vi "HandleObservationSync_003.vi"(8 "error in (no error)":errorcluster, 11 "S4GUI in":refnum<class "S4GUI.lvclass">) -> (0 "error out":errorcluster, 3 "S4GUI out":refnum<class "S4GUI.lvclass">)   [LabVIEW 2018, in "S4GUI.lvclass"] (continued)
          n765 = call-dynamic "Read AcquisitionC.vi"("error in (no error)"=w1948, "S4ACS_GUI in"=w1947) -> ("error out"=w1927:errorcluster, "Acquisition.lvclass"=w1928:refnum<class "Acquisition.lvclass">, "S4ACS_GUI out"=w1952:refnum<class "S4GUI.lvclass">)  [unwired: 7 in]
          n766 = call "Read connection.vi"("error in (no error)"=w1927, "Server in"=w1928) -> ("error out"=w1926:errorcluster, "connection"=w1924:bool, "Server out"=w1925:refnum<class "Acquisition.lvclass">)  [unwired: 7 in]
          n767 = case shown="True" w1924 {
            tunnel: w1925 -> [w1995 w2011]
            tunnel: w1926 -> [w1994 w2010]
            tunnel: [w1995 w2008] -> w1923
            tunnel: [w1994 w2007] -> w1922
            tunnel: [0 ("State") w1997] -> w1898
            frame False {
            }
            frame True {
              n768 = call-dynamic "Read Channel.vi"("error in (no error)"=w2010, "Acquisition in"=w2011) -> ("error out"=w2006:errorcluster, "Channel.lvclass"=w2005:refnum<class "Channel.lvclass">, "Acquisition out"=w2009:refnum<class "Acquisition.lvclass">)  [unwired: 7 in]
              n769 = call-dynamic "Read State Machine.vi"("error in (no error)"=w2006, "Device in"=w2005) -> ("error out"=w1999:errorcluster, "State Machine.lvclass"=w2001:refnum<class "State Machine.lvclass">, "Device out"=w2003:refnum<class "Channel.lvclass">)  [unwired: 7 in]
              n770 = call-dynamic "Read State.vi"("error in (no error)"=w1999, "State Machine in"=w2001) -> ("error out"=w1998:errorcluster, "State"=w1997:i32, "State Machine out"=w2000:refnum<class "State Machine.lvclass">)  [unwired: 7 in]
              n771 = call-dynamic "Write State Machine.vi"("error in (no error)"=w1998, "State Machine.lvclass"=w2000, "Device in"=w2003) -> ("error out"=w2002:errorcluster, "Device out"=w2004:refnum<class "Channel.lvclass">)  [unwired: 7 in]
              n772 = call-dynamic "Write Channel.vi"("error in (no error)"=w2002, "Channel.lvclass"=w2004, "Acquisition in"=w2009) -> ("error out"=w2007:errorcluster, "Acquisition out"=w2008:refnum<class "Acquisition.lvclass">)  [unwired: 7 in]
            }
          }
          n773 = call-dynamic "Write AcquisitionC.vi"("error in (no error)"=w1922, "Acquisition.lvclass"=w1923, "S4ACS_GUI in"=w1952) -> ("error out"=w1946:errorcluster, "S4ACS_GUI out"=w1945:refnum<class "S4GUI.lvclass">)  [unwired: 7 in]
          n774 = call-dynamic "Read AcquisitionD.vi"("error in (no error)"=w1946, "S4ACS_GUI in"=w1945) -> ("error out"=w1919:errorcluster, "Acquisition.lvclass"=w1921:refnum<class "Acquisition.lvclass">, "S4ACS_GUI out"=w1951:refnum<class "S4GUI.lvclass">)  [unwired: 7 in]
          n775 = call "Read connection.vi"("error in (no error)"=w1919, "Server in"=w1921) -> ("error out"=w1918:errorcluster, "connection"=w1917:bool, "Server out"=w1920:refnum<class "Acquisition.lvclass">)  [unwired: 7 in]
          n776 = case shown="True" w1917 {
            tunnel: w1920 -> [w1977 w1993]
            tunnel: w1918 -> [w1976 w1992]
            tunnel: [w1977 w1990] -> w1916
            tunnel: [w1976 w1989] -> w1915
            tunnel: [0 ("State") w1979] -> w1897
            frame False {
            }
            frame True {
              n777 = call-dynamic "Read Channel.vi"("error in (no error)"=w1992, "Acquisition in"=w1993) -> ("error out"=w1988:errorcluster, "Channel.lvclass"=w1987:refnum<class "Channel.lvclass">, "Acquisition out"=w1991:refnum<class "Acquisition.lvclass">)  [unwired: 7 in]
              n778 = call-dynamic "Read State Machine.vi"("error in (no error)"=w1988, "Device in"=w1987) -> ("error out"=w1981:errorcluster, "State Machine.lvclass"=w1983:refnum<class "State Machine.lvclass">, "Device out"=w1985:refnum<class "Channel.lvclass">)  [unwired: 7 in]
              n779 = call-dynamic "Read State.vi"("error in (no error)"=w1981, "State Machine in"=w1983) -> ("error out"=w1980:errorcluster, "State"=w1979:i32, "State Machine out"=w1982:refnum<class "State Machine.lvclass">)  [unwired: 7 in]
              n780 = call-dynamic "Write State Machine.vi"("error in (no error)"=w1980, "State Machine.lvclass"=w1982, "Device in"=w1985) -> ("error out"=w1984:errorcluster, "Device out"=w1986:refnum<class "Channel.lvclass">)  [unwired: 7 in]
              n781 = call-dynamic "Write Channel.vi"("error in (no error)"=w1984, "Channel.lvclass"=w1986, "Acquisition in"=w1991) -> ("error out"=w1989:errorcluster, "Acquisition out"=w1990:refnum<class "Acquisition.lvclass">)  [unwired: 7 in]
            }
          }
          n782 = call-dynamic "Write AcquisitionD.vi"("error in (no error)"=w1915, "Acquisition.lvclass"=w1916, "S4ACS_GUI in"=w1951) -> ("error out"=w1944:errorcluster, "S4ACS_GUI out"=w1909:refnum<class "S4GUI.lvclass">)  [unwired: 7 in]
          n783 = Equal?(x=w1901, y=w1900) -> (x = y?=w1905:bool)
          n784 = Equal?(x=w1910, y=w1900) -> (x = y?=w1914:bool)
          n785 = Equal?(x=w1901, y=w1899) -> (x = y?=w1904:bool)
          n786 = Equal?(x=w1910, y=w1899) -> (x = y?=w1913:bool)
          n787 = Equal?(x=w1901, y=w1898) -> (x = y?=w1903:bool)
          n788 = Equal?(x=w1910, y=w1898) -> (x = y?=w1912:bool)
          n789 = Equal?(x=w1901, y=w1897) -> (x = y?=w1902:bool)
          n790 = Equal?(x=w1910, y=w1897) -> (x = y?=w1911:bool)
          n791 = Compound Arithmetic op=ADD(w1900, w1899, w1898, w1897) -> (w1908:i32)
          n792 = Compound Arithmetic op=OR(w1905, w1904, w1903, w1902) -> (w1895:bool)
          n793 = Compound Arithmetic op=OR(w1914, w1913, w1912, w1911) -> (w1896:bool)
          n794 = Build Array(w1896, w1895) -> (w1894:bool[])
          n795 = Boolean Array To Number(Boolean array=w1894) -> (number=w1893:u32)
          n796 = case shown="0, Default" w1893 {
            tunnel: w1909 -> [w1959 w1967 w1971 w1975]
            tunnel: [w1958 w1966 w1970 w1974] -> w1906
            tunnel: w1908 -> [w1963 _ _ _]
            tunnel: w1907 -> [w1960 _ _ _]
            frame 0, Default {
              n797 = Equal To 0?(x=w1963) -> (x = 0?=w1962:bool)
              n798 = Select(t=u32 360, s=w1962, f=w1960) -> (s? t:f=w1957:u32)
              n799 = Bundle By Name(cluster=w1959, "Obs_state"=w1957) -> (w1958:refnum<class "S4GUI.lvclass">)
            }
            frame 1 {
              n800 = Bundle By Name(cluster=w1967, "Obs_state"=u32 1, "Error Msg"="ERROR: Some channel initialization failed. S4GUI:HandleObservationSync.vi state 272.") -> (w1966:refnum<class "S4GUI.lvclass">)
            }
            frame 2 {
              n801 = Bundle By Name(cluster=w1971, "Obs_state"=u32 1, "Error Msg"="ERROR: Some channel with invalid Exposition Time. S4GUI:HandleObservationSync.vi state 272.") -> (w1970:refnum<class "S4GUI.lvclass">)
            }
            frame 3 {
              n802 = Bundle By Name(cluster=w1975, "Obs_state"=u32 1, "Error Msg"="ERROR: Invalid configuration in the channels. S4GUI:HandleObservationSync.vi state 272.") -> (w1974:refnum<class "S4GUI.lvclass">)
            }
          }
        }
        frame 299 {
          # "Verifcando iniciação dos CICLO:"
          # "T= todos os canais ativos estão zerados."
          # "Exemplo de erro em \"Cycles_done\":\nchA; cycles_done=0; CCD_STATUS=ACTIVE;                                           Seqs_done=15;\nchA; cycles_done=0; CCD_STATUS=IDLE;                                                Seqs_done=16;   =>mudança de seq. com mesmo ciclo\nchA; cycles_done=1; CCD_STATUS=WAITING_EXPOSE_COMMAND; Seqs_done=0;\n\nchB; cycles_done=0; CCD_STATUS=ACTIVE;                                           Seqs_done=15;\nchB; cycles_done=1; CCD_STATUS=WAITING_EXPOSE_COMMAND; Seqs_done=0;     => mudança de seq com novo ciclo"
          # "T=canais receberam STOP"
          # "T= Todos os canais ativos no mesmo ciclo;\nF= Canais em ciclo diferente."
          # "Todos os CYCLES_DONE \nestão zerados?\nSe sim, vai para 327."
          # "Exemplo:\nSET #CYCLES 3\nSET #SEQ 4\ntotal de sequencias: 3 x 4 = 12\n\nseq.        CYCLES_DONE           SEQS_DONE\n1a.                     0                                 0\n2a.                     0                                 1 \n3a.                     0                                 2 \n4a.                     0                                 3 \n                          1                                 4\n5a.                     1                                 0 \n6a.                     1                                 1 \n7a.                     1                                 2 \n8a.                     1                                 3 \n                          2                                 4\n9a.                     2                                 0 \n10a.                   2                                 1 \n11a.                   2                                 2 \n12a.                   2                                 3 \n\nfim                    3                                 4"
          n803 = call-dynamic "Read AcquisitionA.vi"("error in (no error)"=w2100, "S4ACS_GUI in"=w2066) -> ("error out"=w2081:errorcluster, "Acquisition.lvclass"=w2082:refnum<class "Acquisition.lvclass">, "S4ACS_GUI out"=w2102:refnum<class "S4GUI.lvclass">)  [unwired: 7 in]
          n804 = call-dynamic "Read enabled.vi"("error in (no error)"=w2081, "Server in"=w2082) -> ("error out"=w2080:errorcluster, "enabled"=w2061:bool, "Server out"=w2079:refnum<class "Acquisition.lvclass">)  [unwired: 7 in]
          n805 = case shown="True" w2061 {
            tunnel: w2080 -> [w2192 w2208]
            tunnel: [w2193 w2206] -> w2103
            tunnel: [w2192 w2205] -> w2101
            tunnel: [u32 0 ("SequesDone") w2204] -> _
            tunnel: w2079 -> [w2193 w2203]
            tunnel: [TRUE w2202] -> w2065
            tunnel: [FALSE ("stopping") w2195] -> w2057
            frame False {
            }
            frame True {
              # "CYCLES_DONE = 0 ?"
              n806 = call-dynamic "Read Channel.vi"("error in (no error)"=w2208, "Acquisition in"=w2203) -> ("error out"=w2200:errorcluster, "Channel.lvclass"=w2201:refnum<class "Channel.lvclass">, "Acquisition out"=w2207:refnum<class "Acquisition.lvclass">)  [unwired: 7 in]
              n807 = call-dynamic "Read CyclesDone.vi"("error in (no error)"=w2200, "Channel in"=w2201) -> ("error out"=w2198:errorcluster, "CyclesDone"=w2204:u32, "Channel out"=w2199:refnum<class "Channel.lvclass">)  [unwired: 7 in]
              n808 = Equal?(x=w2204, y=u32 0) -> (x = y?=w2202:bool)
              n809 = call-dynamic "Read stopping.vi"("error in (no error)"=w2198, "Channel in"=w2199) -> ("error out"=w2197:errorcluster, "stopping"=w2195:bool, "Channel out"=w2196:refnum<class "Channel.lvclass">)  [unwired: 7 in]
              n810 = call-dynamic "Write Channel.vi"("error in (no error)"=w2197, "Channel.lvclass"=w2196, "Acquisition in"=w2207) -> ("error out"=w2205:errorcluster, "Acquisition out"=w2206:refnum<class "Acquisition.lvclass">)  [unwired: 7 in]
            }
          }
          n811 = call-dynamic "Write AcquisitionA.vi"("error in (no error)"=w2101, "Acquisition.lvclass"=w2103, "S4ACS_GUI in"=w2102) -> ("error out"=w2098:errorcluster, "S4ACS_GUI out"=w2097:refnum<class "S4GUI.lvclass">)  [unwired: 7 in]
          n812 = call "Read AcquisitionB.vi"("error in (no error)"=w2098, "S4ACS_GUI in"=w2097) -> ("error out"=w2075:errorcluster, "Acquisition.lvclass"=w2078:refnum<class "Acquisition.lvclass">, "S4ACS_GUI out"=w2099:refnum<class "S4GUI.lvclass">)  [unwired: 7 in]
          n813 = call-dynamic "Read enabled.vi"("error in (no error)"=w2075, "Server in"=w2078) -> ("error out"=w2076:errorcluster, "enabled"=w2060:bool, "Server out"=w2077:refnum<class "Acquisition.lvclass">)  [unwired: 7 in]
          n814 = case shown="True" w2060 {
            tunnel: w2076 -> [w2172 w2188]
            tunnel: w2077 -> [w2173 w2187]
            tunnel: [u32 0 ("SequesDone") w2182] -> _
            tunnel: [w2172 w2186] -> w2096
            tunnel: [w2173 w2185] -> w2095
            tunnel: [TRUE w2181] -> w2064
            tunnel: [FALSE ("stopping") w2175] -> w2056
            frame False {
            }
            frame True {
              n815 = call-dynamic "Read Channel.vi"("error in (no error)"=w2188, "Acquisition in"=w2187) -> ("error out"=w2179:errorcluster, "Channel.lvclass"=w2180:refnum<class "Channel.lvclass">, "Acquisition out"=w2183:refnum<class "Acquisition.lvclass">)  [unwired: 7 in]
              n816 = call-dynamic "Read CyclesDone.vi"("error in (no error)"=w2179, "Channel in"=w2180) -> ("error out"=w2177:errorcluster, "CyclesDone"=w2182:u32, "Channel out"=w2184:refnum<class "Channel.lvclass">)  [unwired: 7 in]
              n817 = Equal?(x=w2182, y=u32 0) -> (x = y?=w2181:bool)
              n818 = call-dynamic "Read stopping.vi"("error in (no error)"=w2177, "Channel in"=w2184) -> ("error out"=w2176:errorcluster, "stopping"=w2175:bool, "Channel out"=w2178:refnum<class "Channel.lvclass">)  [unwired: 7 in]
              n819 = call-dynamic "Write Channel.vi"("error in (no error)"=w2176, "Channel.lvclass"=w2178, "Acquisition in"=w2183) -> ("error out"=w2186:errorcluster, "Acquisition out"=w2185:refnum<class "Acquisition.lvclass">)  [unwired: 7 in]
            }
          }
          n820 = call "Write AcquisitionB.vi"("error in (no error)"=w2096, "Acquisition.lvclass"=w2095, "S4ACS_GUI in"=w2099) -> ("error out"=w2088:errorcluster, "S4ACS_GUI out"=w2087:refnum<class "S4GUI.lvclass">)  [unwired: 7 in]
          n821 = call-dynamic "Read AcquisitionC.vi"("error in (no error)"=w2088, "S4ACS_GUI in"=w2087) -> ("error out"=w2072:errorcluster, "Acquisition.lvclass"=w2074:refnum<class "Acquisition.lvclass">, "S4ACS_GUI out"=w2090:refnum<class "S4GUI.lvclass">)  [unwired: 7 in]
          n822 = call-dynamic "Read enabled.vi"("error in (no error)"=w2072, "Server in"=w2074) -> ("error out"=w2071:errorcluster, "enabled"=w2059:bool, "Server out"=w2073:refnum<class "Acquisition.lvclass">)  [unwired: 7 in]
          n823 = case shown="True" w2059 {
            tunnel: [w2152 w2168] -> w2091
            tunnel: [w2153 w2167] -> w2089
            tunnel: w2071 -> [w2152 w2164]
            tunnel: w2073 -> [w2153 w2165]
            tunnel: [u32 0 ("SequesDone") w2163] -> _
            tunnel: [TRUE w2162] -> w2063
            tunnel: [FALSE ("stopping") w2155] -> w2055
            frame False {
            }
            frame True {
              n824 = call-dynamic "Read Channel.vi"("error in (no error)"=w2164, "Acquisition in"=w2165) -> ("error out"=w2159:errorcluster, "Channel.lvclass"=w2160:refnum<class "Channel.lvclass">, "Acquisition out"=w2166:refnum<class "Acquisition.lvclass">)  [unwired: 7 in]
              n825 = call-dynamic "Read CyclesDone.vi"("error in (no error)"=w2159, "Channel in"=w2160) -> ("error out"=w2157:errorcluster, "CyclesDone"=w2163:u32, "Channel out"=w2161:refnum<class "Channel.lvclass">)  [unwired: 7 in]
              n826 = Equal?(x=w2163, y=u32 0) -> (x = y?=w2162:bool)
              n827 = call-dynamic "Read stopping.vi"("error in (no error)"=w2157, "Channel in"=w2161) -> ("error out"=w2156:errorcluster, "stopping"=w2155:bool, "Channel out"=w2158:refnum<class "Channel.lvclass">)  [unwired: 7 in]
              n828 = call-dynamic "Write Channel.vi"("error in (no error)"=w2156, "Channel.lvclass"=w2158, "Acquisition in"=w2166) -> ("error out"=w2168:errorcluster, "Acquisition out"=w2167:refnum<class "Acquisition.lvclass">)  [unwired: 7 in]
            }
          }
          n829 = call-dynamic "Write AcquisitionC.vi"("error in (no error)"=w2091, "Acquisition.lvclass"=w2089, "S4ACS_GUI in"=w2090) -> ("error out"=w2085:errorcluster, "S4ACS_GUI out"=w2086:refnum<class "S4GUI.lvclass">)  [unwired: 7 in]
          n830 = call-dynamic "Read AcquisitionD.vi"("error in (no error)"=w2085, "S4ACS_GUI in"=w2086) -> ("error out"=w2068:errorcluster, "Acquisition.lvclass"=w2070:refnum<class "Acquisition.lvclass">, "S4ACS_GUI out"=w2092:refnum<class "S4GUI.lvclass">)  [unwired: 7 in]
          n831 = call-dynamic "Read enabled.vi"("error in (no error)"=w2068, "Server in"=w2070) -> ("error out"=w2067:errorcluster, "enabled"=w2058:bool, "Server out"=w2069:refnum<class "Acquisition.lvclass">)  [unwired: 7 in]
          n832 = case shown="True" w2058 {
            tunnel: [w2133 w2148] -> w2094
            tunnel: [w2132 w2147] -> w2093
            tunnel: w2069 -> [w2133 w2146]
            tunnel: w2067 -> [w2132 w2145]
            tunnel: [u32 0 ("SequesDone") w2143] -> _
            tunnel: [TRUE w2142] -> w2062
            tunnel: [FALSE ("stopping") w2135] -> w2054
            frame False {
            }
            frame True {
              n833 = call-dynamic "Read Channel.vi"("error in (no error)"=w2145, "Acquisition in"=w2146) -> ("error out"=w2139:errorcluster, "Channel.lvclass"=w2140:refnum<class "Channel.lvclass">, "Acquisition out"=w2144:refnum<class "Acquisition.lvclass">)  [unwired: 7 in]
              n834 = call-dynamic "Read CyclesDone.vi"("error in (no error)"=w2139, "Channel in"=w2140) -> ("error out"=w2137:errorcluster, "CyclesDone"=w2143:u32, "Channel out"=w2141:refnum<class "Channel.lvclass">)  [unwired: 7 in]
              n835 = Equal?(x=w2143, y=u32 0) -> (x = y?=w2142:bool)
              n836 = call-dynamic "Read stopping.vi"("error in (no error)"=w2137, "Channel in"=w2141) -> ("error out"=w2136:errorcluster, "stopping"=w2135:bool, "Channel out"=w2138:refnum<class "Channel.lvclass">)  [unwired: 7 in]
              n837 = call-dynamic "Write Channel.vi"("error in (no error)"=w2136, "Channel.lvclass"=w2138, "Acquisition in"=w2144) -> ("error out"=w2147:errorcluster, "Acquisition out"=w2148:refnum<class "Acquisition.lvclass">)  [unwired: 7 in]
            }
          }
          n838 = Compound Arithmetic op=AND(w2065, w2064, w2063, w2062) -> (w2051:bool)
          n839 = Compound Arithmetic op=OR(w2057, w2056, w2055, w2054) -> (w2053:bool)
          n840 = call-dynamic "Write AcquisitionD.vi"("error in (no error)"=w2093, "Acquisition.lvclass"=w2094, "S4ACS_GUI in"=w2092) -> ("error out"=w2083:errorcluster, "S4ACS_GUI out"=w2084:refnum<class "S4GUI.lvclass">)  [unwired: 7 in]
          n841 = case shown="True" w2051 {
            tunnel: w2084 -> [w2114 w2125]
            tunnel: [w2113 w2124] -> w2052
            tunnel: w2053 -> [_ w2123]
            tunnel: w2050 -> [_ w2120]
            frame False {
              # "Esperando todos os canais habilitados mudarem de cyclesDone.\nE verificando a maior duracao de cubo entre os canais."
              n842 = local read "time307"() -> (w2112:u32)
              n843 = Tick Count (ms)() -> (millisecond timer value=w2111:u32)
              n844 = Subtract(x=w2111, y=w2112) -> (x-y=w2107:u32)
              n845 = call-dynamic "GetGreatestCube.vi"("S4GUI in"=w2114) -> ("S4GUI out"=w2109:refnum<class "S4GUI.lvclass">, "greatest (ms)"=w2105:dbl)  [unwired: 8 in, 1 out]
              n846 = To Double Precision Float(number=w2107) -> (double precision float=w2110:dbl)
              n847 = Add(x=1000.0 ("y"), y=w2105) -> (x+y=w2104:dbl)
              n848 = Less?(x=w2104, y=w2110) -> (x < y?=w2108:bool)
              n849 = case shown="True" w2108 {
                tunnel: w2109 -> [w2115 w2119]
                tunnel: [w2115 w2118] -> w2113
                frame False {
                }
                frame True {
                  n850 = Bundle By Name(cluster=w2119, "Obs_state"=u32 1, "Error Msg"="ERROR: Cycles_Done reseting timeout. - HandleObservationSync.vi state 299.") -> (w2118:refnum<class "S4GUI.lvclass">)
                }
              }
            }
            frame True {
              # "STOP?"
              n851 = case shown="False" w2123 {
                tunnel: [w2126 u32 0] -> w2122
                tunnel: w2120 -> [w2127 _]
                frame False {
                  n852 = Increment(x=w2127) -> (x+1=w2126:u32)
                }
                frame True {
                }
              }
              n853 = Bundle By Name(cluster=w2125, "Obs_state"=w2122, "cyclesDone"=u32 0) -> (w2124:refnum<class "S4GUI.lvclass">)
            }
          }
        }
        frame 300 {
          # "Verifica se é modo fotometria ou polarimetria:\nTrue = polarimetria (esatdo 301)\nFalse = fotometria (estado 321)"
          n854 = flat-sequence {
            tunnel: w2213 -> [w2226]
            tunnel: [w2226] -> w2212
            frame #0 {
              n855 = local read "time3"() -> (w2228:u32)
              n856 = local read "time4"() -> (w2225:u32)
              n857 = Tick Count (ms)() -> (millisecond timer value=w2224:u32)
              n858 = Subtract(x=w2225, y=w2228) -> (x-y=→"delay 3-4":u32)
              n859 = local write "time1"(w2224) -> ()
            }
          }
          n860 = call "Read Instrument.lvclass.vi"("error in (no error)"=w2212, "S4ACS_GUI in"=w2223) -> ("error out"=w2218:errorcluster, "Instrument.lvclass"=w2219:refnum<class "Instrument.lvclass">, "S4ACS_GUI out"=w2217:refnum<class "S4GUI.lvclass">)  [unwired: 7 in]
          n861 = call-dynamic "Read mode.vi"("error in (no error)"=w2218, "Instrument in"=w2219) -> ("error out"=w2214:errorcluster, "mode"=w2216:bool)  [unwired: 7 in, 1 out]
          n862 = Select(t=u32 301, s=w2216, f=u32 321 ("t")) -> (s? t:f=w2221:u32)
          n863 = Bundle By Name(cluster=w2217, "Obs_state"=w2221, "cyclesDone"=u32 0, "sequesDone"=u32 0, "seqAtual"=u32 0) -> (w2222:refnum<class "S4GUI.lvclass">)
        }
        frame 301 {
          # "Configurando para ACS esperar comando EXPOSE"
          n864 = call-dynamic "Read AcquisitionA.vi"("error in (no error)"=w2291, "S4ACS_GUI in"=w2292) -> ("error out"=w2246:errorcluster, "Acquisition.lvclass"=w2247:refnum<class "Acquisition.lvclass">, "S4ACS_GUI out"=w2294:refnum<class "S4GUI.lvclass">)  [unwired: 7 in]
          n865 = call-dynamic "Read enabled.vi"("error in (no error)"=w2246, "Server in"=w2247) -> ("error out"=w2245:errorcluster, "enabled"=w2232:bool, "Server out"=w2248:refnum<class "Acquisition.lvclass">)  [unwired: 7 in]
          n866 = call "Read connection.vi"("error in (no error)"=w2245, "Server in"=w2248) -> ("error out"=w2271:errorcluster, "connection"=w2255:bool, "Server out"=w2272:refnum<class "Acquisition.lvclass">)  [unwired: 7 in]
          n867 = And(x=w2255, y=w2232) -> (x .and. y?=w2256:bool)
          n868 = case shown="True" w2256 {
            tunnel: w2272 -> [w2409 w2428]
            tunnel: w2271 -> [w2408 w2427]
            tunnel: [w2409 w2425] -> w2295
            tunnel: [w2408 w2424] -> w2293
            tunnel: [w2405 u32 0 ("New_State")] -> w2261
            tunnel: w2232 -> [w2404 _]
            frame False {
              n869 = Select(t=u32 1, s=w2404, f=u32 0) -> (s? t:f=w2405:u32)
            }
            frame True {
              n870 = call-dynamic "Read Channel.vi"("error in (no error)"=w2427, "Acquisition in"=w2428) -> ("error out"=w2411:errorcluster, "Channel.lvclass"=w2414:refnum<class "Channel.lvclass">, "Acquisition out"=w2426:refnum<class "Acquisition.lvclass">)  [unwired: 7 in]
              n871 = call-dynamic "Write wait_expose.vi"("error in (no error)"=w2411, "wait_expose"=TRUE, "Channel in"=w2414) -> ("error out"=w2410:errorcluster, "Channel out"=w2413:refnum<class "Channel.lvclass">)  [unwired: 7 in]
              n872 = call-dynamic "Read State Machine.vi"("error in (no error)"=w2410, "Device in"=w2413) -> ("error out"=w2421:errorcluster, "State Machine.lvclass"=w2423:refnum<class "State Machine.lvclass">, "Device out"=w2419:refnum<class "Channel.lvclass">)  [unwired: 7 in]
              n873 = call "Next State.vi"("error in (no error)"=w2421, "New_State"=40, "State Machine in"=w2423) -> ("error out"=w2416:errorcluster, "State Machine out"=w2417:refnum<class "State Machine.lvclass">)  [unwired: 7 in]
              n874 = call-dynamic "Write State Machine.vi"("error in (no error)"=w2416, "State Machine.lvclass"=w2417, "Device in"=w2419) -> ("error out"=w2418:errorcluster, "Device out"=w2420:refnum<class "Channel.lvclass">)  [unwired: 7 in]
              n875 = call-dynamic "Write Channel.vi"("error in (no error)"=w2418, "Channel.lvclass"=w2420, "Acquisition in"=w2426) -> ("error out"=w2424:errorcluster, "Acquisition out"=w2425:refnum<class "Acquisition.lvclass">)  [unwired: 7 in]
            }
          }
          n876 = call-dynamic "Write AcquisitionA.vi"("error in (no error)"=w2293, "Acquisition.lvclass"=w2295, "S4ACS_GUI in"=w2294) -> ("error out"=w2288:errorcluster, "S4ACS_GUI out"=w2289:refnum<class "S4GUI.lvclass">)  [unwired: 7 in]
          n877 = call "Read AcquisitionB.vi"("error in (no error)"=w2288, "S4ACS_GUI in"=w2289) -> ("error out"=w2242:errorcluster, "Acquisition.lvclass"=w2244:refnum<class "Acquisition.lvclass">, "S4ACS_GUI out"=w2286:refnum<class "S4GUI.lvclass">)  [unwired: 7 in]
          n878 = call-dynamic "Read enabled.vi"("error in (no error)"=w2242, "Server in"=w2244) -> ("error out"=w2241:errorcluster, "enabled"=w2231:bool, "Server out"=w2243:refnum<class "Acquisition.lvclass">)  [unwired: 7 in]
          n879 = call "Read connection.vi"("error in (no error)"=w2241, "Server in"=w2243) -> ("error out"=w2269:errorcluster, "connection"=w2253:bool, "Server out"=w2270:refnum<class "Acquisition.lvclass">)  [unwired: 7 in]
          n880 = And(x=w2253, y=w2231) -> (x .and. y?=w2254:bool)
          n881 = case shown="True" w2254 {
            tunnel: w2270 -> [w2384 w2403]
            tunnel: w2269 -> [w2383 w2402]
            tunnel: [w2384 w2400] -> w2287
            tunnel: [w2383 w2399] -> w2285
            tunnel: [w2380 u32 0 ("New_State")] -> w2260
            tunnel: w2231 -> [w2379 _]
            frame False {
              n882 = Select(t=u32 2, s=w2379, f=u32 0) -> (s? t:f=w2380:u32)
            }
            frame True {
              n883 = call-dynamic "Read Channel.vi"("error in (no error)"=w2402, "Acquisition in"=w2403) -> ("error out"=w2386:errorcluster, "Channel.lvclass"=w2388:refnum<class "Channel.lvclass">, "Acquisition out"=w2401:refnum<class "Acquisition.lvclass">)  [unwired: 7 in]
              n884 = call-dynamic "Write wait_expose.vi"("error in (no error)"=w2386, "wait_expose"=TRUE, "Channel in"=w2388) -> ("error out"=w2385:errorcluster, "Channel out"=w2387:refnum<class "Channel.lvclass">)  [unwired: 7 in]
              n885 = call-dynamic "Read State Machine.vi"("error in (no error)"=w2385, "Device in"=w2387) -> ("error out"=w2396:errorcluster, "State Machine.lvclass"=w2398:refnum<class "State Machine.lvclass">, "Device out"=w2394:refnum<class "Channel.lvclass">)  [unwired: 7 in]
              n886 = call "Next State.vi"("error in (no error)"=w2396, "New_State"=40, "State Machine in"=w2398) -> ("error out"=w2391:errorcluster, "State Machine out"=w2392:refnum<class "State Machine.lvclass">)  [unwired: 7 in]
              n887 = call-dynamic "Write State Machine.vi"("error in (no error)"=w2391, "State Machine.lvclass"=w2392, "Device in"=w2394) -> ("error out"=w2393:errorcluster, "Device out"=w2395:refnum<class "Channel.lvclass">)  [unwired: 7 in]
              n888 = call-dynamic "Write Channel.vi"("error in (no error)"=w2393, "Channel.lvclass"=w2395, "Acquisition in"=w2401) -> ("error out"=w2399:errorcluster, "Acquisition out"=w2400:refnum<class "Acquisition.lvclass">)  [unwired: 7 in]
            }
          }
          n889 = call "Write AcquisitionB.vi"("error in (no error)"=w2285, "Acquisition.lvclass"=w2287, "S4ACS_GUI in"=w2286) -> ("error out"=w2281:errorcluster, "S4ACS_GUI out"=w2280:refnum<class "S4GUI.lvclass">)  [unwired: 7 in]
          n890 = call-dynamic "Read AcquisitionC.vi"("error in (no error)"=w2281, "S4ACS_GUI in"=w2280) -> ("error out"=w2238:errorcluster, "Acquisition.lvclass"=w2240:refnum<class "Acquisition.lvclass">, "S4ACS_GUI out"=w2283:refnum<class "S4GUI.lvclass">)  [unwired: 7 in]
          n891 = call-dynamic "Read enabled.vi"("error in (no error)"=w2238, "Server in"=w2240) -> ("error out"=w2237:errorcluster, "enabled"=w2230:bool, "Server out"=w2239:refnum<class "Acquisition.lvclass">)  [unwired: 7 in]
          n892 = call "Read connection.vi"("error in (no error)"=w2237, "Server in"=w2239) -> ("error out"=w2267:errorcluster, "connection"=w2250:bool, "Server out"=w2268:refnum<class "Acquisition.lvclass">)  [unwired: 7 in]
          n893 = And(x=w2250, y=w2230) -> (x .and. y?=w2252:bool)
          n894 = case shown="True" w2252 {
            tunnel: [w2358 w2372] -> w2284
            tunnel: [w2359 w2371] -> w2282
            tunnel: w2268 -> [w2359 w2369]
            tunnel: w2267 -> [w2358 w2368]
            tunnel: [w2355 u32 0 ("New_State")] -> w2259
            tunnel: w2230 -> [w2354 _]
            frame False {
              n895 = Select(t=u32 4, s=w2354, f=u32 0) -> (s? t:f=w2355:u32)
            }
            frame True {
              n896 = call-dynamic "Read Channel.vi"("error in (no error)"=w2368, "Acquisition in"=w2369) -> ("error out"=w2361:errorcluster, "Channel.lvclass"=w2363:refnum<class "Channel.lvclass">, "Acquisition out"=w2370:refnum<class "Acquisition.lvclass">)  [unwired: 7 in]
              n897 = call-dynamic "Write wait_expose.vi"("error in (no error)"=w2361, "wait_expose"=TRUE, "Channel in"=w2363) -> ("error out"=w2360:errorcluster, "Channel out"=w2362:refnum<class "Channel.lvclass">)  [unwired: 7 in]
              n898 = call-dynamic "Read State Machine.vi"("error in (no error)"=w2360, "Device in"=w2362) -> ("error out"=w2375:errorcluster, "State Machine.lvclass"=w2373:refnum<class "State Machine.lvclass">, "Device out"=w2377:refnum<class "Channel.lvclass">)  [unwired: 7 in]
              n899 = call "Next State.vi"("error in (no error)"=w2375, "New_State"=40, "State Machine in"=w2373) -> ("error out"=w2367:errorcluster, "State Machine out"=w2366:refnum<class "State Machine.lvclass">)  [unwired: 7 in]
              n900 = call-dynamic "Write State Machine.vi"("error in (no error)"=w2367, "State Machine.lvclass"=w2366, "Device in"=w2377) -> ("error out"=w2378:errorcluster, "Device out"=w2376:refnum<class "Channel.lvclass">)  [unwired: 7 in]
              n901 = call-dynamic "Write Channel.vi"("error in (no error)"=w2378, "Channel.lvclass"=w2376, "Acquisition in"=w2370) -> ("error out"=w2372:errorcluster, "Acquisition out"=w2371:refnum<class "Acquisition.lvclass">)  [unwired: 7 in]
            }
          }
          n902 = call-dynamic "Write AcquisitionC.vi"("error in (no error)"=w2284, "Acquisition.lvclass"=w2282, "S4ACS_GUI in"=w2283) -> ("error out"=w2278:errorcluster, "S4ACS_GUI out"=w2277:refnum<class "S4GUI.lvclass">)  [unwired: 7 in]
          n903 = call-dynamic "Read AcquisitionD.vi"("error in (no error)"=w2278, "S4ACS_GUI in"=w2277) -> ("error out"=w2234:errorcluster, "Acquisition.lvclass"=w2236:refnum<class "Acquisition.lvclass">, "S4ACS_GUI out"=w2276:refnum<class "S4GUI.lvclass">)  [unwired: 7 in]
          n904 = call-dynamic "Read enabled.vi"("error in (no error)"=w2234, "Server in"=w2236) -> ("error out"=w2233:errorcluster, "enabled"=w2229:bool, "Server out"=w2235:refnum<class "Acquisition.lvclass">)  [unwired: 7 in]
          n905 = call "Read connection.vi"("error in (no error)"=w2233, "Server in"=w2235) -> ("error out"=w2265:errorcluster, "connection"=w2249:bool, "Server out"=w2266:refnum<class "Acquisition.lvclass">)  [unwired: 7 in]
          n906 = And(x=w2249, y=w2229) -> (x .and. y?=w2251:bool)
          n907 = case shown="True" w2251 {
            tunnel: w2265 -> [w2333 w2353]
            tunnel: [w2333 w2352] -> w2279
            tunnel: w2266 -> [w2334 w2345]
            tunnel: [w2334 w2343] -> w2275
            tunnel: [w2330 u32 0 ("New_State")] -> w2258
            tunnel: w2229 -> [w2329 _]
            frame False {
              n908 = Select(t=u32 8, s=w2329, f=u32 0) -> (s? t:f=w2330:u32)
            }
            frame True {
              n909 = call-dynamic "Read Channel.vi"("error in (no error)"=w2353, "Acquisition in"=w2345) -> ("error out"=w2335:errorcluster, "Channel.lvclass"=w2338:refnum<class "Channel.lvclass">, "Acquisition out"=w2344:refnum<class "Acquisition.lvclass">)  [unwired: 7 in]
              n910 = call-dynamic "Write wait_expose.vi"("error in (no error)"=w2335, "wait_expose"=TRUE, "Channel in"=w2338) -> ("error out"=w2336:errorcluster, "Channel out"=w2337:refnum<class "Channel.lvclass">)  [unwired: 7 in]
              n911 = call-dynamic "Read State Machine.vi"("error in (no error)"=w2336, "Device in"=w2337) -> ("error out"=w2349:errorcluster, "State Machine.lvclass"=w2351:refnum<class "State Machine.lvclass">, "Device out"=w2347:refnum<class "Channel.lvclass">)  [unwired: 7 in]
              n912 = call "Next State.vi"("error in (no error)"=w2349, "New_State"=40, "State Machine in"=w2351) -> ("error out"=w2341:errorcluster, "State Machine out"=w2342:refnum<class "State Machine.lvclass">)  [unwired: 7 in]
              n913 = call-dynamic "Write State Machine.vi"("error in (no error)"=w2341, "State Machine.lvclass"=w2342, "Device in"=w2347) -> ("error out"=w2346:errorcluster, "Device out"=w2348:refnum<class "Channel.lvclass">)  [unwired: 7 in]
              n914 = call-dynamic "Write Channel.vi"("error in (no error)"=w2346, "Channel.lvclass"=w2348, "Acquisition in"=w2344) -> ("error out"=w2352:errorcluster, "Acquisition out"=w2343:refnum<class "Acquisition.lvclass">)  [unwired: 7 in]
            }
          }
          n915 = call-dynamic "Write AcquisitionD.vi"("error in (no error)"=w2279, "Acquisition.lvclass"=w2275, "S4ACS_GUI in"=w2276) -> ("error out"=w2274:errorcluster, "S4ACS_GUI out"=w2273:refnum<class "S4GUI.lvclass">)  [unwired: 7 in]
          n916 = Compound Arithmetic op=ADD(w2261, w2260, w2259, w2258) -> (w2262:u32)
          n917 = case shown="0, Default" w2262 {
            tunnel: w2257 -> [w2298 _ _ _ _ _ _ _ _ _ _ _ _ _ _ _]
            tunnel: [w2297 u32 1 ("Obs_state") u32 1 ("Obs_state") u32 1 ("Obs_state") u32 1 ("Obs_state") u32 1 ("Obs_state") u32 1 ("Obs_state") u32 1 ("Obs_state") u32 1 ("Obs_state") u32 1 ("Obs_state") u32 1 ("Obs_state") u32 1 ("Obs_state") u32 1 ("Obs_state") u32 1 ("Obs_state") u32 1 ("Obs_state") u32 1 ("Obs_state")] -> w2263
            tunnel: ["" ("Error Msg") "ERROR: Lost channel 1 connection... - HandleObservationSync.vi state 301" ("Error Msg") "ERROR: Lost channel 2 connection...- HandleObservationSync.vi state 301" ("Error Msg") "ERROR: Lost channels 1 and 2 connection...- HandleObservationSync.vi state 301" ("Error Msg") "ERROR: Lost channel 3 connection...- HandleObservationSync.vi state 301" ("Error Msg") "ERROR: Lost channels 1 and  3 connection...- HandleObservationSync.vi state 301" ("Error Msg") "ERROR:  Lost channels 2 and  3 connection...- HandleObservationSync.vi state 301" ("Error Msg") "ERROR:  Lost channels 1, 2 and  3 connection...- HandleObservationSync.vi state 301" ("Error Msg") "ERROR: Lost channel 4 connection...- HandleObservationSync.vi state 301" ("Error Msg") "ERROR:  Lost channels 1 and 4 connection...- HandleObservationSync.vi state 301" ("Error Msg") "ERROR:  Lost channels 2 and 4 connection...- HandleObservationSync.vi state 301" ("Error Msg") "ERROR: Lost channels 1, 2 and 4 connection...- HandleObservationSync.vi state 301" ("Error Msg") "ERROR: Lost channels 3 and 4 connection...- HandleObservationSync.vi state 301" ("Error Msg") "ERROR: Lost channels 1, 3 and 4 connection...- HandleObservationSync.vi state 301" ("Error Msg") "ERROR: Lost channels 2, 3 and 4 connection...- HandleObservationSync.vi state 301" ("Error Msg") "ERROR: Lost channels 1, 2, 3 and 4 connection...- HandleObservationSync.vi state 301" ("Error Msg")] -> w2264
            frame 0, Default {
              n918 = Increment(x=w2298) -> (x+1=w2297:u32)
            }
            frame 1 {
            }
            frame 2 {
            }
            frame 3 {
            }
            frame 4 {
            }
            frame 5 {
            }
            frame 6 {
            }
            frame 7 {
            }
            frame 8 {
            }
            frame 9 {
            }
            frame 10 {
            }
            frame 11 {
            }
            frame 12 {
            }
            frame 13 {
            }
            frame 14 {
            }
            frame 15 {
            }
          }
          n919 = Bundle By Name(cluster=w2273, "Obs_state"=w2263, "Error Msg"=w2264) -> (w2290:refnum<class "S4GUI.lvclass">)
        }
        frame 302 {
          # "Espera terminar o envio de WAIT EXPOSE COMMAND para todos os ACS."
          n920 = call-dynamic "VerifyAcqIdle.vi"("error in (no error)"=w2430, "S4GUI in"=w2429) -> ("error out"=w2435:errorcluster, "idle"=w2434:bool, "S4GUI out"=w2436:refnum<class "S4GUI.lvclass">)  [unwired: 7 in]
          n921 = Increment(x=w2432) -> (x+1=w2431:u32)
          n922 = Select(t=w2431, s=w2434, f=w2432) -> (s? t:f=w2433:u32)
          n923 = Bundle By Name(cluster=w2436, "Obs_state"=w2433) -> (w2437:refnum<class "S4GUI.lvclass">)
        }
        frame 303 {
          n924 = flat-sequence {
            tunnel: w2443 -> [w2482]
            tunnel: [w2482] -> w2442
            frame #0 {
              n925 = Tick Count (ms)() -> (millisecond timer value=→"time1":u32)
            }
          }
          n926 = call "Read Instrument.lvclass.vi"("error in (no error)"=w2442, "S4ACS_GUI in"=w2478) -> ("error out"=w2480:errorcluster, "Instrument.lvclass"=w2481:refnum<class "Instrument.lvclass">, "S4ACS_GUI out"=w2439:refnum<class "S4GUI.lvclass">)  [unwired: 7 in]
          n927 = call "Read WPROT.vi"("error in (no error)"=w2480, "Instrument in"=w2481) -> ("error out"=w2471:errorcluster, "Opt_Selector.lvclass"=w2472:refnum<class "Opt_Selector.lvclass">, "Instrument out"=w2479:refnum<class "Instrument.lvclass">)  [unwired: 7 in]
          n928 = call-dynamic "getTargetPos.vi"("error in (no error)"=w2471, "Opt_Selector in"=w2472) -> ("error out"=w2470:errorcluster, "Target Pos"=w2450:u16, "Opt_Selector out"=w2469:refnum<class "Opt_Selector.lvclass">)  [unwired: 7 in]
          n929 = Unbundle By Name(w2439) -> ("seqAtual"=w2441:u32)
          n930 = Build Array(-1.0 ("element"), 0.0 ("element"), 22.5 ("element"), 45.0 ("element"), 67.5 ("element"), 90.0 ("element"), 112.5 ("element"), 135.0 ("element"), 157.5 ("element"), 180.0 ("element"), 202.5 ("element"), 225.0 ("element"), 247.5 ("element"), 270.0 ("element"), 292.5 ("element"), 315.0 ("element"), 337.5 ("element")) -> (w2462:dbl[])
          n931 = Index Array(array=w2462, index=w2450) -> (element=w2449:dbl)
          n932 = case shown="0, Default" w2450 {
            selector: w2450 -> [_ w2516]
            tunnel: w2479 -> [w2492 w2504]
            tunnel: [w2492 w2504] -> w2445
            tunnel: [w2489 w2503] -> w2444
            tunnel: w2475 -> [_ w2518]
            tunnel: [u32 314 w2517] -> w2474
            tunnel: w2470 -> [w2490 w2512]
            tunnel: w2469 -> [w2491 w2511]
            tunnel: w2449 -> [_ w2506]
            tunnel: [w2487 w2505] -> w2446
            tunnel: [u32 0 w2494] -> w2440
            tunnel: w2441 -> [_ w2495]
            frame 0, Default {
              # "Terminou uma sequência.\nRecupera as posições em SEQ e desvia para 314 para verificar se há mais ciclos."
              # "Recupera a sequencia anterior para o caso \nde repetição da sequencia (sem precisar clicar \nnas posicoes desejadas novamente)."
              n933 = call-dynamic "Read sequencia_ant.vi"("error in (no error)"=w2490, "Opt_Selector in"=w2491) -> ("error out"=w2486:errorcluster, "sequencia_ant"=w2485:u16, "Opt_Selector out"=w2488:refnum<class "Opt_Selector.lvclass">)  [unwired: 7 in]
              n934 = call-dynamic "Write sequencia.vi"("error in (no error)"=w2486, "sequencia"=w2485, "Opt_Selector in"=w2488) -> ("error out"=w2489:errorcluster, "Opt_Selector out"=w2487:refnum<class "Opt_Selector.lvclass">)  [unwired: 7 in]
            }
            frame 1..16 {
              # "Inicia o Ticks com\nvalor do relogio atual"
              # "Espera até 40 x 0.25s (= 10s) para\nmecanismo entrar em READY"
              n935 = Number To Decimal String(number=w2516) -> (decimal integer string=w2515:string)  [unwired: 1 in]
              n936 = Concatenate Strings("WP" ("string"), w2515) -> (w2513:string)
              n937 = call "Write target name.vi"("error in (no error)"=w2512, "target name"=w2513, "Optics in"=w2511) -> ("error out"=w2509:errorcluster, "Optics out"=w2510:refnum<class "Opt_Selector.lvclass">)  [unwired: 7 in]
              n938 = call "Write target.vi"("error in (no error)"=w2509, "target"=w2506, "Optics in"=w2510) -> ("error out"=w2508:errorcluster, "Optics out"=w2507:refnum<class "Opt_Selector.lvclass">)  [unwired: 7 in]
              n939 = call-dynamic "Read State Machine.vi"("error in (no error)"=w2508, "Device in"=w2507) -> ("error out"=w2520:errorcluster, "State Machine.lvclass"=w2522:refnum<class "State Machine.lvclass">, "Device out"=w2519:refnum<class "Opt_Selector.lvclass">)  [unwired: 7 in]
              n940 = Increment(x=w2518) -> (x+1=w2517:u32)
              n941 = call "Next State.vi"("error in (no error)"=w2520, "New_State"=1, "State Machine in"=w2522) -> ("error out"=w2501:errorcluster, "State Machine out"=w2502:refnum<class "State Machine.lvclass">)  [unwired: 7 in]
              n942 = Increment(x=w2495) -> (x+1=w2494:u32)
              n943 = call-dynamic "Write Timer.vi"("error in (no error)"=w2501, "Timer"=u32 40, "State Machine in"=w2502) -> ("error out"=w2498:errorcluster, "State Machine out"=w2499:refnum<class "State Machine.lvclass">)  [unwired: 7 in]
              n944 = call-dynamic "Init Ticks2.vi"("error in (no error)"=w2498, "State Machine in"=w2499) -> ("error out"=w2497:errorcluster, "State Machine out"=w2496:refnum<class "State Machine.lvclass">)  [unwired: 8 in]
              n945 = call-dynamic "Write State Machine.vi"("error in (no error)"=w2497, "State Machine.lvclass"=w2496, "Device in"=w2519) -> ("error out"=w2503:errorcluster, "Device out"=w2505:refnum<class "Opt_Selector.lvclass">)  [unwired: 7 in]
            }
          }
          n946 = Bundle By Name(cluster=w2439, "seqAtual"=w2440) -> (w2438:refnum<class "S4GUI.lvclass">)
          n947 = call "Write WPROT.vi"("error in (no error)"=w2444, "Opt_Selector.lvclass"=w2446, "Instrument in"=w2445) -> ("error out"=w2448:errorcluster, "Instrument out"=w2447:refnum<class "Instrument.lvclass">)  [unwired: 7 in]
          n948 = call "Write Instrument.lvclass.vi"("error in (no error)"=w2448, "Instrument.lvclass"=w2447, "S4ACS_GUI in"=w2438) -> ("error out"=w2477:errorcluster, "S4ACS_GUI out"=w2476:refnum<class "S4GUI.lvclass">)  [unwired: 7 in]
          n949 = Bundle By Name(cluster=w2476, "Obs_state"=w2474) -> (w2473:refnum<class "S4GUI.lvclass">)
        }
        frame 304 {
          # "Espera terminar o movimento da lamina para disparar a aquisição\ndos canais ativos.\n\nOV 20230424: Não precisa mais atualizar o valor de WPPOS com o\ncomando WRITE_HEADER porque o ACS já recebeu a sequência de\nposições da lâmina."
          n950 = flat-sequence {
            tunnel: w2549 -> [w2574]
            tunnel: [w2574] -> w2548
            frame #0 {
              n951 = Tick Count (ms)() -> (millisecond timer value=w2573:u32)
              "time 2" <- w2573
              n952 = local read "time1"() -> (w2572:u32)
              n953 = Subtract(x=w2573, y=w2572) -> (x-y=→"delay wp":u32)
            }
          }
          n954 = call "Read Instrument.lvclass.vi"("error in (no error)"=w2548, "S4ACS_GUI in"=w2556) -> ("error out"=w2561:errorcluster, "Instrument.lvclass"=w2562:refnum<class "Instrument.lvclass">, "S4ACS_GUI out"=w2558:refnum<class "S4GUI.lvclass">)  [unwired: 7 in]
          n955 = call "Read WPROT.vi"("error in (no error)"=w2561, "Instrument in"=w2562) -> ("error out"=w2555:errorcluster, "Opt_Selector.lvclass"=w2554:refnum<class "Opt_Selector.lvclass">, "Instrument out"=w2560:refnum<class "Instrument.lvclass">)  [unwired: 7 in]
          n956 = call-dynamic "Read State Machine.vi"("error in (no error)"=w2555, "Device in"=w2554) -> ("error out"=w2529:errorcluster, "State Machine.lvclass"=w2532:refnum<class "State Machine.lvclass">, "Device out"=w2552:refnum<class "Opt_Selector.lvclass">)  [unwired: 7 in]
          n957 = call-dynamic "Verif Clock 2.vi"("error in (no error)"=w2529, "period (ms)"=u32 20000 ("period"), "State Machine in"=w2532) -> ("error out"=w2528:errorcluster, "time elapsed"=→"time elapsed":u32, "State Machine out"=w2531:refnum<class "State Machine.lvclass">)  [unwired: 6 in]
          n958 = call-dynamic "Read Timeout 2.vi"("error in (no error)"=w2528, "State Machine in"=w2531) -> ("error out"=w2527:errorcluster, "Timeout 2"=w2535:bool, "State Machine out"=w2530:refnum<class "State Machine.lvclass">)  [unwired: 7 in]
          n959 = call-dynamic "Read State.vi"("error in (no error)"=w2527, "State Machine in"=w2530) -> ("error out"=w2546:errorcluster, "State"=w2550:i32, "State Machine out"=w2547:refnum<class "State Machine.lvclass">)  [unwired: 7 in]
          n960 = Equal To 0?(x=w2550) -> (x = 0?=w2538:bool)
          n961 = call-dynamic "Write State Machine.vi"("error in (no error)"=w2546, "State Machine.lvclass"=w2547, "Device in"=w2552) -> ("error out"=w2551:errorcluster, "Device out"=w2553:refnum<class "Opt_Selector.lvclass">)  [unwired: 7 in]
          n962 = call "Write WPROT.vi"("error in (no error)"=w2551, "Opt_Selector.lvclass"=w2553, "Instrument in"=w2560) -> ("error out"=w2557:errorcluster, "Instrument out"=w2559:refnum<class "Instrument.lvclass">)  [unwired: 7 in]
          n963 = call "Write Instrument.lvclass.vi"("error in (no error)"=w2557, "Instrument.lvclass"=w2559, "S4ACS_GUI in"=w2558) -> ("error out"=w2537:errorcluster, "S4ACS_GUI out"=w2526:refnum<class "S4GUI.lvclass">)  [unwired: 7 in]
          n964 = case shown="True" w2535 {
            tunnel: w2534 -> [w2564 _]
            tunnel: [w2564 u32 1 ("Obs_state")] -> w2533
            tunnel: w2526 -> [w2563 w2568]
            tunnel: [w2563 w2567] -> w2525
            frame False {
            }
            frame True {
              n965 = Bundle By Name(cluster=w2568, "Error Msg"="ERROR: moving waveplate timeout  (S4GUI:HandleObservationSync.vi - state 302)") -> (w2567:refnum<class "S4GUI.lvclass">)
            }
          }
          n966 = Unbundle By Name(w2526) -> ("cyclesDone"=w2542:u32, "seqAtual"=w2541:u32)
          n967 = Decrement(x=w2541) -> (x-1=w2523:u32)
          n968 = Add(x=w2542, y=w2523) -> (x+y=w2540:u32)
          n969 = Equal To 0?(x=w2540) -> (x = 0?=w2543:bool)
          n970 = case shown="True" w2543 {
            tunnel: [u32 308 ("t") u32 308 ("t")] -> w2544
            frame False {
              (unwired) u32 310 ("t")
              # "Não é 1a seq:\nvai direto para\nenvio do trigger"
            }
            frame True {
              # "1a sequencia:\nenvia EXPOSE"
            }
          }
          n971 = Select(t=w2544, s=w2538, f=w2533) -> (s? t:f=w2545:u32)
          n972 = Bundle By Name(cluster=w2525, "Obs_state"=w2545) -> (w2539:refnum<class "S4GUI.lvclass">)
        }
        frame 308 {
          n973 = call-dynamic "Read AcquisitionA.vi"("error in (no error)"=w2637, "S4ACS_GUI in"=w2638) -> ("error out"=w2592:errorcluster, "Acquisition.lvclass"=w2593:refnum<class "Acquisition.lvclass">, "S4ACS_GUI out"=w2640:refnum<class "S4GUI.lvclass">)  [unwired: 7 in]
          n974 = call-dynamic "Read enabled.vi"("error in (no error)"=w2592, "Server in"=w2593) -> ("error out"=w2591:errorcluster, "enabled"=w2578:bool, "Server out"=w2594:refnum<class "Acquisition.lvclass">)  [unwired: 7 in]
          n975 = call "Read connection.vi"("error in (no error)"=w2591, "Server in"=w2594) -> ("error out"=w2617:errorcluster, "connection"=w2601:bool, "Server out"=w2618:refnum<class "Acquisition.lvclass">)  [unwired: 7 in]
          n976 = And(x=w2601, y=w2578) -> (x .and. y?=w2602:bool)
          n977 = case shown="True" w2602 {
            tunnel: w2618 -> [w2747 w2763]
            tunnel: w2617 -> [w2746 w2762]
            tunnel: [w2747 w2760] -> w2641
            tunnel: [w2746 w2759] -> w2639
            tunnel: [w2743 u32 0 ("New_State")] -> w2607
            tunnel: w2578 -> [w2742 _]
            frame False {
              n978 = Select(t=u32 1, s=w2742, f=u32 0) -> (s? t:f=w2743:u32)
            }
            frame True {
              n979 = call-dynamic "Read Channel.vi"("error in (no error)"=w2762, "Acquisition in"=w2763) -> ("error out"=w2755:errorcluster, "Channel.lvclass"=w2754:refnum<class "Channel.lvclass">, "Acquisition out"=w2761:refnum<class "Acquisition.lvclass">)  [unwired: 7 in]
              n980 = call-dynamic "Read State Machine.vi"("error in (no error)"=w2755, "Device in"=w2754) -> ("error out"=w2756:errorcluster, "State Machine.lvclass"=w2758:refnum<class "State Machine.lvclass">, "Device out"=w2752:refnum<class "Channel.lvclass">)  [unwired: 7 in]
              n981 = call "Next State.vi"("error in (no error)"=w2756, "New_State"=50, "State Machine in"=w2758) -> ("error out"=w2749:errorcluster, "State Machine out"=w2750:refnum<class "State Machine.lvclass">)  [unwired: 7 in]
              n982 = call-dynamic "Write State Machine.vi"("error in (no error)"=w2749, "State Machine.lvclass"=w2750, "Device in"=w2752) -> ("error out"=w2751:errorcluster, "Device out"=w2753:refnum<class "Channel.lvclass">)  [unwired: 7 in]
              n983 = call-dynamic "Write Channel.vi"("error in (no error)"=w2751, "Channel.lvclass"=w2753, "Acquisition in"=w2761) -> ("error out"=w2759:errorcluster, "Acquisition out"=w2760:refnum<class "Acquisition.lvclass">)  [unwired: 7 in]
            }
          }
          n984 = call-dynamic "Write AcquisitionA.vi"("error in (no error)"=w2639, "Acquisition.lvclass"=w2641, "S4ACS_GUI in"=w2640) -> ("error out"=w2634:errorcluster, "S4ACS_GUI out"=w2635:refnum<class "S4GUI.lvclass">)  [unwired: 7 in]
          n985 = call "Read AcquisitionB.vi"("error in (no error)"=w2634, "S4ACS_GUI in"=w2635) -> ("error out"=w2588:errorcluster, "Acquisition.lvclass"=w2590:refnum<class "Acquisition.lvclass">, "S4ACS_GUI out"=w2632:refnum<class "S4GUI.lvclass">)  [unwired: 7 in]
          n986 = call-dynamic "Read enabled.vi"("error in (no error)"=w2588, "Server in"=w2590) -> ("error out"=w2587:errorcluster, "enabled"=w2577:bool, "Server out"=w2589:refnum<class "Acquisition.lvclass">)  [unwired: 7 in]
          n987 = call "Read connection.vi"("error in (no error)"=w2587, "Server in"=w2589) -> ("error out"=w2615:errorcluster, "connection"=w2599:bool, "Server out"=w2616:refnum<class "Acquisition.lvclass">)  [unwired: 7 in]
          n988 = And(x=w2599, y=w2577) -> (x .and. y?=w2600:bool)
          n989 = case shown="True" w2600 {
            tunnel: w2616 -> [w2725 w2741]
            tunnel: w2615 -> [w2724 w2740]
            tunnel: [w2725 w2738] -> w2633
            tunnel: [w2724 w2737] -> w2631
            tunnel: [w2721 u32 0 ("New_State")] -> w2606
            tunnel: w2577 -> [w2720 _]
            frame False {
              n990 = Select(t=u32 2, s=w2720, f=u32 0) -> (s? t:f=w2721:u32)
            }
            frame True {
              n991 = call-dynamic "Read Channel.vi"("error in (no error)"=w2740, "Acquisition in"=w2741) -> ("error out"=w2733:errorcluster, "Channel.lvclass"=w2732:refnum<class "Channel.lvclass">, "Acquisition out"=w2739:refnum<class "Acquisition.lvclass">)  [unwired: 7 in]
              n992 = call-dynamic "Read State Machine.vi"("error in (no error)"=w2733, "Device in"=w2732) -> ("error out"=w2734:errorcluster, "State Machine.lvclass"=w2736:refnum<class "State Machine.lvclass">, "Device out"=w2730:refnum<class "Channel.lvclass">)  [unwired: 7 in]
              n993 = call "Next State.vi"("error in (no error)"=w2734, "New_State"=50, "State Machine in"=w2736) -> ("error out"=w2727:errorcluster, "State Machine out"=w2728:refnum<class "State Machine.lvclass">)  [unwired: 7 in]
              n994 = call-dynamic "Write State Machine.vi"("error in (no error)"=w2727, "State Machine.lvclass"=w2728, "Device in"=w2730) -> ("error out"=w2729:errorcluster, "Device out"=w2731:refnum<class "Channel.lvclass">)  [unwired: 7 in]
              n995 = call-dynamic "Write Channel.vi"("error in (no error)"=w2729, "Channel.lvclass"=w2731, "Acquisition in"=w2739) -> ("error out"=w2737:errorcluster, "Acquisition out"=w2738:refnum<class "Acquisition.lvclass">)  [unwired: 7 in]
            }
          }
          n996 = call "Write AcquisitionB.vi"("error in (no error)"=w2631, "Acquisition.lvclass"=w2633, "S4ACS_GUI in"=w2632) -> ("error out"=w2627:errorcluster, "S4ACS_GUI out"=w2626:refnum<class "S4GUI.lvclass">)  [unwired: 7 in]
          n997 = call-dynamic "Read AcquisitionC.vi"("error in (no error)"=w2627, "S4ACS_GUI in"=w2626) -> ("error out"=w2584:errorcluster, "Acquisition.lvclass"=w2586:refnum<class "Acquisition.lvclass">, "S4ACS_GUI out"=w2629:refnum<class "S4GUI.lvclass">)  [unwired: 7 in]
          n998 = call-dynamic "Read enabled.vi"("error in (no error)"=w2584, "Server in"=w2586) -> ("error out"=w2583:errorcluster, "enabled"=w2576:bool, "Server out"=w2585:refnum<class "Acquisition.lvclass">)  [unwired: 7 in]
          n999 = call "Read connection.vi"("error in (no error)"=w2583, "Server in"=w2585) -> ("error out"=w2613:errorcluster, "connection"=w2596:bool, "Server out"=w2614:refnum<class "Acquisition.lvclass">)  [unwired: 7 in]
          n1000 = And(x=w2596, y=w2576) -> (x .and. y?=w2598:bool)
          n1001 = case shown="True" w2598 {
            tunnel: [w2702 w2711] -> w2630
            tunnel: [w2703 w2710] -> w2628
            tunnel: w2614 -> [w2703 w2708]
            tunnel: w2613 -> [w2702 w2707]
            tunnel: [w2699 u32 0 ("New_State")] -> w2605
            tunnel: w2576 -> [w2698 _]
            frame False {
              n1002 = Select(t=u32 4, s=w2698, f=u32 0) -> (s? t:f=w2699:u32)
            }
            frame True {
              n1003 = call-dynamic "Read Channel.vi"("error in (no error)"=w2707, "Acquisition in"=w2708) -> ("error out"=w2715:errorcluster, "Channel.lvclass"=w2716:refnum<class "Channel.lvclass">, "Acquisition out"=w2709:refnum<class "Acquisition.lvclass">)  [unwired: 7 in]
              n1004 = call-dynamic "Read State Machine.vi"("error in (no error)"=w2715, "Device in"=w2716) -> ("error out"=w2714:errorcluster, "State Machine.lvclass"=w2712:refnum<class "State Machine.lvclass">, "Device out"=w2718:refnum<class "Channel.lvclass">)  [unwired: 7 in]
              n1005 = call "Next State.vi"("error in (no error)"=w2714, "New_State"=50, "State Machine in"=w2712) -> ("error out"=w2706:errorcluster, "State Machine out"=w2705:refnum<class "State Machine.lvclass">)  [unwired: 7 in]
              n1006 = call-dynamic "Write State Machine.vi"("error in (no error)"=w2706, "State Machine.lvclass"=w2705, "Device in"=w2718) -> ("error out"=w2719:errorcluster, "Device out"=w2717:refnum<class "Channel.lvclass">)  [unwired: 7 in]
              n1007 = call-dynamic "Write Channel.vi"("error in (no error)"=w2719, "Channel.lvclass"=w2717, "Acquisition in"=w2709) -> ("error out"=w2711:errorcluster, "Acquisition out"=w2710:refnum<class "Acquisition.lvclass">)  [unwired: 7 in]
            }
          }
          n1008 = call-dynamic "Write AcquisitionC.vi"("error in (no error)"=w2630, "Acquisition.lvclass"=w2628, "S4ACS_GUI in"=w2629) -> ("error out"=w2624:errorcluster, "S4ACS_GUI out"=w2623:refnum<class "S4GUI.lvclass">)  [unwired: 7 in]
          n1009 = call-dynamic "Read AcquisitionD.vi"("error in (no error)"=w2624, "S4ACS_GUI in"=w2623) -> ("error out"=w2580:errorcluster, "Acquisition.lvclass"=w2582:refnum<class "Acquisition.lvclass">, "S4ACS_GUI out"=w2622:refnum<class "S4GUI.lvclass">)  [unwired: 7 in]
          n1010 = call-dynamic "Read enabled.vi"("error in (no error)"=w2580, "Server in"=w2582) -> ("error out"=w2579:errorcluster, "enabled"=w2575:bool, "Server out"=w2581:refnum<class "Acquisition.lvclass">)  [unwired: 7 in]
          n1011 = call "Read connection.vi"("error in (no error)"=w2579, "Server in"=w2581) -> ("error out"=w2611:errorcluster, "connection"=w2595:bool, "Server out"=w2612:refnum<class "Acquisition.lvclass">)  [unwired: 7 in]
          n1012 = And(x=w2595, y=w2575) -> (x .and. y?=w2597:bool)
          n1013 = case shown="True" w2597 {
            tunnel: w2611 -> [w2680 w2697]
            tunnel: [w2680 w2696] -> w2625
            tunnel: w2612 -> [w2681 w2687]
            tunnel: [w2681 w2685] -> w2621
            tunnel: [w2677 u32 0 ("New_State")] -> w2604
            tunnel: w2575 -> [w2676 _]
            frame False {
              n1014 = Select(t=u32 8, s=w2676, f=u32 0) -> (s? t:f=w2677:u32)
            }
            frame True {
              n1015 = call-dynamic "Read Channel.vi"("error in (no error)"=w2697, "Acquisition in"=w2687) -> ("error out"=w2692:errorcluster, "Channel.lvclass"=w2691:refnum<class "Channel.lvclass">, "Acquisition out"=w2686:refnum<class "Acquisition.lvclass">)  [unwired: 7 in]
              n1016 = call-dynamic "Read State Machine.vi"("error in (no error)"=w2692, "Device in"=w2691) -> ("error out"=w2693:errorcluster, "State Machine.lvclass"=w2695:refnum<class "State Machine.lvclass">, "Device out"=w2689:refnum<class "Channel.lvclass">)  [unwired: 7 in]
              n1017 = call "Next State.vi"("error in (no error)"=w2693, "New_State"=50, "State Machine in"=w2695) -> ("error out"=w2683:errorcluster, "State Machine out"=w2684:refnum<class "State Machine.lvclass">)  [unwired: 7 in]
              n1018 = call-dynamic "Write State Machine.vi"("error in (no error)"=w2683, "State Machine.lvclass"=w2684, "Device in"=w2689) -> ("error out"=w2688:errorcluster, "Device out"=w2690:refnum<class "Channel.lvclass">)  [unwired: 7 in]
              n1019 = call-dynamic "Write Channel.vi"("error in (no error)"=w2688, "Channel.lvclass"=w2690, "Acquisition in"=w2686) -> ("error out"=w2696:errorcluster, "Acquisition out"=w2685:refnum<class "Acquisition.lvclass">)  [unwired: 7 in]
            }
          }
